vi "solar_app Quit.vi"(8 "error in (no error)":errorcluster) -> (0 "error out":errorcluster)   [LabVIEW 2018]
doc: "This VI updates the Configs Directory depending on the system setups defined in the main target's configuration file. A system setup appends a sub-directory to the Configs Dir for different application configurations."
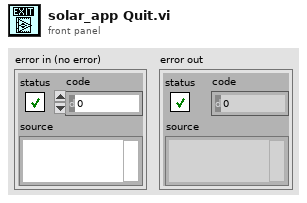
[diagram p1: front panel]
types:
  T1 = enum32{"invalid app kind", "Development System", "Run Time System", "Student Edition", "Embedded LabVIEW", "Evaluation", "Custom"}
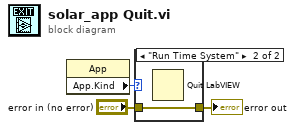
[diagram p0: block diagram]
diagram:
  n1 = property on="Property Node" class="App"() -> ("App.Kind"=w3:T1)  [unwired: 2 in, 2 out]
  n2 = case shown="\"Run Time System\"" w3 {
    tunnel: [w4 w5] -> w2
    tunnel: "error in (no error)" -> [w4 w5]
    frame Default {
    }
    frame "Run Time System" {
      n3 = Quit LabVIEW() -> ()  [unwired: 1 in]
    }
  }
  "error out" <- w2
